vi "Read Value.vi"(8 "error in (no error)":errorcluster caption="entrée d'erreur (pas d'erreur)", 11 "DAQmxTaskDOutput_Emulate en entrée":refnum<class "DAQmxTaskDOutput_Emulate.lvclass">) -> (0 "error out":errorcluster caption="sortie d'erreur", 1 "Data":bool, 2 "Data string":string, 3 "DAQmxTaskDOutput_Emulate en sortie":refnum<class "DAQmxTaskDOutput_Emulate.lvclass">)   [LabVIEW 2018, in "DAQmxTaskDOutput_Emulate.lvclass"]
uses:
  DAQmxTaskDOutput_Emulate.lvclass
  C:/Users/Sergey Denisov/Documents/REPS/TRANCON/Classes/DAQmxTasks/DAQmxTask.lvclass
  DAQmxTask.lvclass/DAQmxTask.ctl
  DAQmxTask.lvclass
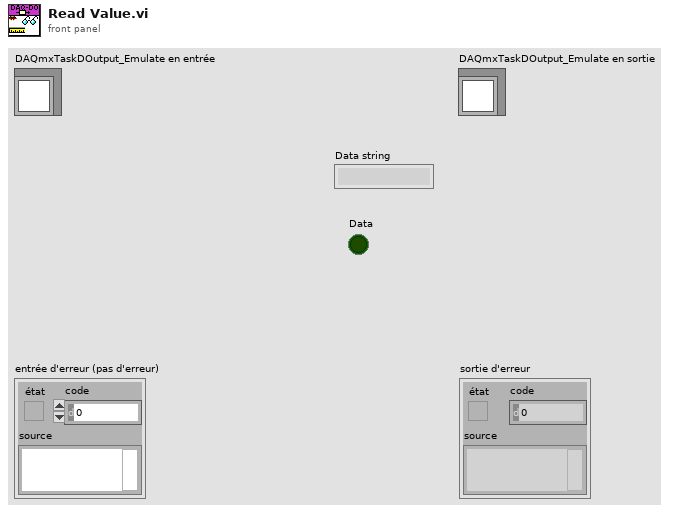
[diagram p1: front panel]
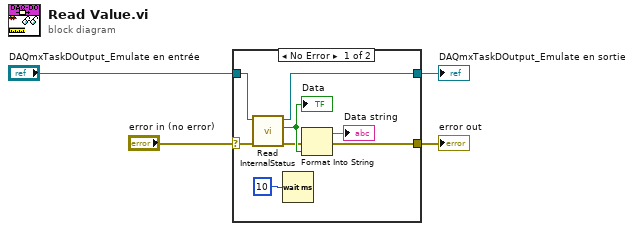
[diagram p0: block diagram]
diagram:
  n1 = case shown="No Error" "error in (no error)" {
    selector: "error in (no error)" -> [w8 w13]
    tunnel: [w6 w14] -> w3
    tunnel: "DAQmxTaskDOutput_Emulate en entrée" -> [w9 w14]
    tunnel: [w12 w13] -> w1
    frame No Error {
      n2 = call "Read InternalStatus.vi"("error in (no error)"=w8, "DAQmxTask in"=w9) -> ("error out"=w5:errorcluster, "InternalStatus"=w7:bool, "DAQmxTask out"=w6:refnum<class "DAQmxTaskDOutput_Emulate.lvclass">)  [unwired: 7 in]
      "Data" <- w7
      n3 = Wait (ms)(milliseconds to wait=u32 10) -> ()  [unwired: 1 out]
      n4 = Format Into String(error in=w5, w7) -> (resulting string=→"Data string":string, error out=w12:errorcluster)  [unwired: 2 in]
    }
    frame Error {
    }
  }
  "error out" <- w1
  "DAQmxTaskDOutput_Emulate en sortie" <- w3
